vi "claerData.vi"(0 "Real":dbl) -> ()   [LabVIEW 2012]
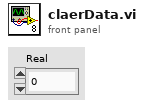
[diagram p1: front panel]
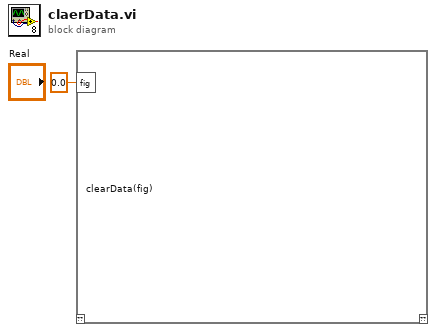
[diagram p0: block diagram]
diagram:
  n1 = script code="clearData(fig)"("fig"=0.0 ("Real")) -> ()  [unwired: 1 in, 1 out]
